vi "Drag Over Draw.vi"(8 "error in (no error)":errorcluster, 10 "DragOver Output":T1={"Displayed Row"=0, "Position"=enum."On Row", "Row's TreeItem index"=0, "indent"=0, "Accepted?"=FALSE, "Insertion index"=0, "Top left visible TreeItem index"=0, "Bar type"=enum."tilda up"}, 11 "BetterHandle in":refnum<class "BetterHandle.lvclass">) -> (0 "error out":errorcluster, 3 "BetterHandle out":refnum<class "BetterHandle.lvclass">)   [LabVIEW 2020, in "BetterDragAndDrop.lvlib" / "BetterHandle.lvclass"]
uses:
  BetterHandle.lvclass
  SubVIs/DragOver Output.ctl
  SubVIs/DragOverPosition.ctl
  BetterTreeBar/SubVIs/Horizontal Bar Enumeration.ctl
  BetterHandle.lvclass/BetterHandle.ctl
  BetterTreeBar/BetterHorizontalBar.lvclass
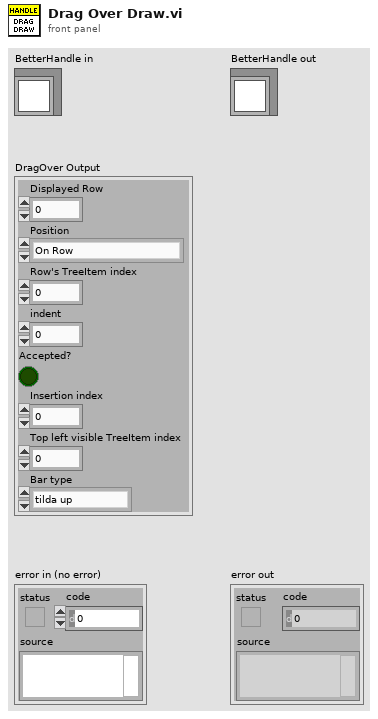
[diagram p1: front panel]
types:
  T1 = typedef "BetterDragAndDrop.lvlib/BetterHandle.lvclass/DragOver Output.ctl" = cluster{"Displayed Row":i32, "Position":T2, "Row's TreeItem index":i32, "indent":i32, "Accepted?":bool, "Insertion index":i32, "Top left visible TreeItem index":i32, "Bar type":T3}
  T2 = typedef "BetterDragAndDrop.lvlib/BetterHandle.lvclass/DragOverPosition.ctl" = enum16{"On Row", "Inbetween"}
  T3 = typedef "BetterDragAndDrop.lvlib/BetterHorizontalBar.lvclass/Horizontal Bar Enumeration.ctl" = enum16{"None", "only bar", "tilda up"}
  T4 = typedef "BetterDragAndDrop.lvlib/BetterHandle.lvclass/Pixel Constants.ctl" = cluster{"Row Header height":i32, "Row height":i32, "Column Header Offset":i32}
  T5 = typedef "LVPositionTypeDef.ctl" = cluster{"Left":i32, "Top":i32}
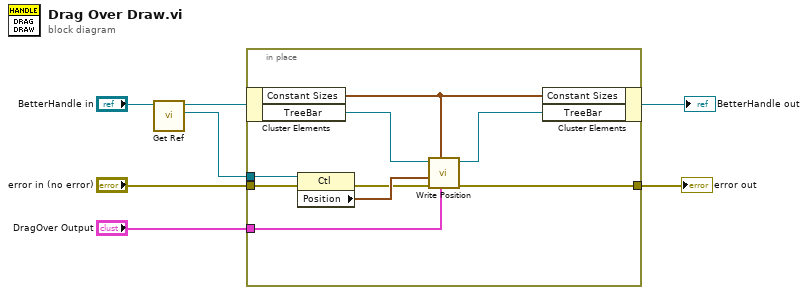
[diagram p0: block diagram]
diagram:
  n1 = call-dynamic "Get Ref.vi"("BetterHandle in"="BetterHandle in") -> ("Tree/LB/MCL ref"=w4:refnum<vi>, "BetterHandle out"=w5:refnum<class "BetterHandle.lvclass">)  [unwired: 8 in, 1 out]
  n2 = in-place {
    in-place-border: w4 -> [w14]
    in-place-border: "DragOver Output" -> [w9]
    in-place-border: "error in (no error)" -> [w11]
    in-place-border: [w10] -> w1
    n3 = in-place-cluster #1(w5) -> ("Constant Sizes"=w8:T4, "TreeBar"=w13:refnum<class "BetterHorizontalBar.lvclass">)
    n4 = property class="Ctl"(reference=w14, error in=w11) -> (error out=w15:errorcluster, "Position"=w16:T5)  [unwired: 1 out]
    n5 = call "Write Position.vi"("DragOver Output"=w9, "Constant Sizes"=w8, "error in (no error)"=w15, "Ref.Position"=w16, "BetterTreeBar in"=w13) -> ("error out"=w10:errorcluster, "BetterTreeBar out"=w12:refnum<class "BetterHorizontalBar.lvclass">)  [unwired: 5 in]
    n6 = in-place-cluster #1("Constant Sizes"=w8, "TreeBar"=w12) -> (→"BetterHandle out":refnum<class "BetterHandle.lvclass">)
  }
  "error out" <- w1
